vi "Configure TSP Link Instrument Node.vi"(7 "Group Number (0)":i32, 8 "error in (no error)":errorcluster, 9 "Node Number (1)":i32=1, 10 "Number Type (0: Node)":i32(ring) items=["Node", "Group"], 11 "VISA resource name":refnum<visa-resource-name>) -> (0 "error out":errorcluster, 3 "VISA resource name out":refnum<visa-resource-name>)   [LabVIEW 2019, in "Keithley 2600 Series.lvlib"]
doc: "Configures the instrument node number and group number.\n\n<b>Note:</b>\nThis VI is not available on the models 2604B, 2614B, and 2634B."
uses:
  Keithley 2600 Series.lvlib
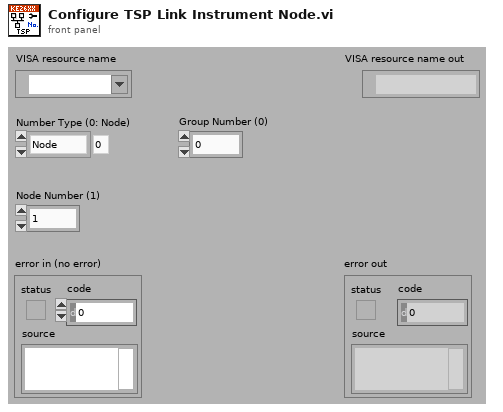
[diagram p1: front panel]
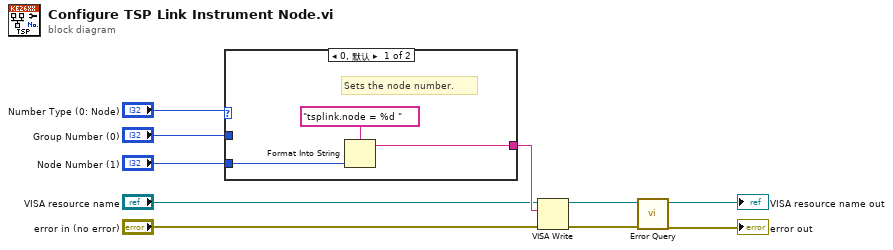
[diagram p0: block diagram]
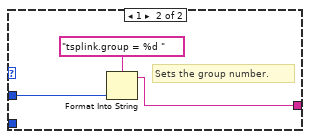
[diagram p2: hidden frame]
diagram:
  n1 = case shown="0, 默认" "Number Type (0: Node)" {
    tunnel: "Group Number (0)" -> [_ w15]
    tunnel: "Node Number (1)" -> [w12 _]
    tunnel: [w11 w14] -> w8
    frame 0, Default {
      # "Sets the node number."
      n2 = Format Into String(format string="tsplink.node = %d ", w12) -> (resulting string=w11:string)  [unwired: 2 in, 1 out]
    }
    frame 1 {
      # "Sets the group number."
      n3 = Format Into String(format string="tsplink.group = %d ", w15) -> (resulting string=w14:string)  [unwired: 2 in, 1 out]
    }
  }
  n4 = VISA Write(VISA resource name="VISA resource name", write buffer=w8, error in (no error)="error in (no error)") -> (VISA resource name out=w5:refnum<visa-resource-name>, error out=w4:errorcluster)  [unwired: 1 out]
  n5 = call "Error Query.vi"("error in (no error)"=w4, "VISA resource name"=w5) -> ("error out"=→"error out":errorcluster, "VISA resource name out"=→"VISA resource name out":refnum<visa-resource-name>)  [unwired: 6 in, 2 out]
